vi "Begin.vi"(8 "error in":errorcluster) -> (0 "error out":errorcluster)   [LabVIEW 2016]
doc: "Called before other user functions, this VI is expected to open initial I/O refnums, load in file data, and do all program initialization. Notice that the <B>error out</B> terminal is simply used for data flow. Wiring it to other structures or subVIs ensures that this VI runs first."
uses:
  <vilib>/Rock Robotics/WPI/DriverStation/WPI_DriverStationRobotMode2.ctl
  <vilib>/Rock Robotics/WPI/Joystick/WPI_JoystickDeviceEnum.ctl
  <vilib>/Rock Robotics/SystemInterfaces/DIO/FPGA_DIOPWMChannel.ctl
  <vilib>/Rock Robotics/SystemInterfaces/AI/FPGA_AIChannel.ctl
  <vilib>/Rock Robotics/SystemInterfaces/DIO/FPGA_DIOChannel.ctl
  <vilib>/Rock Robotics/WPI/Solenoid/WPI_SolenoidChannel.ctl
  <vilib>/Rock Robotics/SystemInterfaces/spilib/spi_bus.ctl
  <vilib>/Rock Robotics/WPI/Solenoid/WPI_SolenoidValue.ctl
  <vilib>/Rock Robotics/WPI/SafetyOutput/WPI_SafetyOutputConfigMenu.ctl
  <vilib>/Rock Robotics/WPI/ThirdParty/CanMotor/TalonSRX/WPI_CANTalonSRX_APIControlMode.ctl
  <vilib>/Rock Robotics/SystemInterfaces/AI/FPGA_AIGyroChannel.ctl
  Robot Global Data.vi
  <vilib>/Rock Robotics/Network Tables/NT Write String Array.vi
  <vilib>/Rock Robotics/WPI/MotorControl/WPI_MotorControlOpen VictorSP.vi
  <vilib>/Rock Robotics/Network Tables/NT Write Number.vi
  <vilib>/Rock Robotics/WPI/Counter/WPI_CounterDigitalInputToDigitalSource.vi
  <vilib>/Rock Robotics/WPI/Solenoid/WPI_SolenoidOpenSingle.vi
  <vilib>/Rock Robotics/WPI/Solenoid/WPI_SolenoidOpenDouble.vi
  <vilib>/Rock Robotics/WPI/Gyro/WPI_GyroXRS450_SPI_Open.vi
  <vilib>/Rock Robotics/WPI/Solenoid/WPI_SolenoidSetEnum.vi
  <vilib>/Rock Robotics/WPI/RobotDrive/WPI_RobotDriveOpen4MotorWithExistingMotors.vi
  <vilib>/Rock Robotics/WPI/Gyro/WPI_GyroAnalogOpen.vi
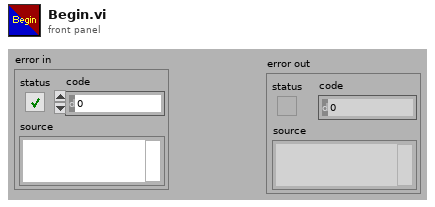
[diagram p1: front panel]
types:
  T1 = typedef "FPGA_AIGyroChannel.ctl" = enum8{"AI 0", "AI 1", "Invalid"}
  T2 = typedef "WPI_CANTalonSRX_APIControlMode.ctl" = enum8{"Percent VBus", "Speed", "Position", "Slave", "Unchanged / Invalid", "Voltage Compensation", "Current", "Motion Profile", "Motion Magic"}
  T3 = typedef "FPGA_DIOPWMChannel.ctl" = enum8{"PWM 0", "PWM 1", "PWM 2", "PWM 3", "PWM 4", "PWM 5", "PWM 6", "PWM 7", "PWM 8", "PWM 9", "PWM MXP 0", "PWM MXP 1", "PWM MXP 2", "PWM MXP 3", "PWM MXP 4", "PWM MXP 5", "PWM MXP 6", "PWM MXP 7", "PWM MXP 8", "PWM MXP 9", "Invalid"}
  T4 = typedef "WPI_SafetyOutputConfigMenu.ctl" = enum16{"Enable", "Disable"}
  T5 = typedef "WPI_SolenoidValue.ctl" = enum16{"Off", "On", "Forward", "Reverse"}
  T6 = typedef "spi_bus.ctl" = enum16{"SPI On-Board, CS0", "SPI On-Board, CS1", "SPI On-Board, CS2", "SPI On-Board, CS3", "SPI MXP", "Invalid"}
  T7 = typedef "WPI_SolenoidChannel.ctl" = enum8{"Solenoid 0", "Solenoid 1", "Solenoid 2", "Solenoid 3", "Solenoid 4", "Solenoid 5", "Solenoid 6", "Solenoid 7", "Invalid"}
  T8 = typedef "FPGA_DIOChannel.ctl" = enum8{"DIO 0", "DIO 1", "DIO 2", "DIO 3", "DIO 4", "DIO 5", "DIO 6", "DIO 7", "DIO 8", "DIO 9", "DIO MXP 0", "DIO MXP 1", "DIO MXP 2", "DIO MXP 3", "DIO MXP 4", "DIO MXP 5", "DIO MXP 6", "DIO MXP 7", "DIO MXP 8", "DIO MXP 9", "DIO MXP 10", "DIO MXP 11", "DIO MXP 12", "DIO MXP 13", "DIO MXP 14", "DIO MXP 15", "SPI Port CS1", "SPI Port CS2", "SPI Port CS3", "SPI Port MISO", "SPI Port MOSI", "Invalid"}
  T9 = typedef "FPGA_AIChannel.ctl" = enum8{"AI 0", "AI 1", "AI 2", "AI 3", "AI MXP 0", "AI MXP 1", "AI MXP 2", "AI MXP 3", "Invalid"}
  T10 = typedef "WPI_JoystickDeviceEnum.ctl" = enum16{"USB 0", "USB 1", "USB 2", "USB 3", "USB 4", "USB 5"}
  T11 = typedef "WPI_DriverStationRobotMode2.ctl" = enum16{"Autonomous Disabled", "Autonomous Enabled", "Teleop Disabled", "Teleop Enabled", "Disconnected", "Finish", "Test Disabled", "Test Enabled", "Emergency Stopped"}
  T12 = typedef "WPI_MotorControlDeviceRef.ctl" = cluster{"DeviceStatus":errorcluster, "Type":T13, "PWM":cluster{"PWM Channel":T3, "DeadBand":T14}, "CAN":cluster{"Device Number":u8, "SetOutput VI Ref":variant, "GetOutput VI Ref":variant, "Enable VI Ref":variant, "Disable VI Ref":variant, "Data":variant}, "Invert":bool}
  T13 = typedef "WPI_MotorControlType.ctl" = enum16{"PWM", "CAN"}
  T14 = typedef "WPI_PWMDeadband.ctl" = cluster{"Name":string, "maxPositivePwm":i32, "minPositivePwm":i32, "centerPwm":i32, "maxNegativePwm":i32, "minNegativePwm":i32, "angularRange":u16}
  T15 = typedef "WPI_PotentiometerDevRef.ctl" = cluster{"DevStatus":errorcluster, "Analog Channel":T9, "Invert Output":bool}
  T16 = typedef "WPI_DigitalInputDevRef.ctl" = cluster{"DevStatus":errorcluster, "DIO Channel":T8}
  T17 = typedef "WPI_JoystickDevRef.ctl" = cluster{"Device":T10}
  T18 = typedef "WPI_SolenoidDevRef.ctl" = cluster{"DevStatus":errorcluster, "Pneumatics Control Module":u8, "Forward Solenoid Channel":T7, "Reverse Solenoid Channel":T7}
  T19 = typedef "WPI_RobotDriveDevRef.ctl" = cluster{"DevStatus":errorcluster, "Motors[]":T12[], "Square Inputs":bool, "Max Output":dbl}
  T20 = typedef "FPGA_CounterEncoderSourceConvertionLVSourceType.ctl" = cluster{"DevStatus":errorcluster, "AnalogTriggerMode?":bool, "DigitalMode":cluster{"DIO Channel":T21}, "AnalogTriggerMode":cluster{"AnalogTriggerIndex":T22, "OutputType":T23}}
  T21 = typedef "FPGA_DIODigitalSourceChannel.ctl" = enum8{"DIO 0", "DIO 1", "DIO 2", "DIO 3", "DIO 4", "DIO 5", "DIO 6", "DIO 7", "DIO 8", "DIO 9", "DIO MXP 0", "DIO MXP 1", "DIO MXP 2", "DIO MXP 3", "DIO MXP 4", "DIO MXP 5", "DIO MXP 6", "DIO MXP 7", "DIO MXP 8", "DIO MXP 9", "DIO MXP 10", "DIO MXP 11", "DIO MXP 12", "DIO MXP 13", "DIO MXP 14", "DIO MXP 15", "Disabled"}
  T22 = typedef "FPGA_AnalogTriggerIndex.ctl" = enum8{"Trig 0", "Trig 1", "Trig 2", "Trig 3", "Trig 4", "Trig 5", "Trig 6", "Trig 7", "Invalid"}
  T23 = typedef "FPGA_AnalogTriggerOutType.ctl" = enum16{"InWindow", "TriggerState", "Rising", "Falling"}
  T24 = typedef "WPI_EncoderDevRef.ctl" = cluster{"DevStatus":errorcluster, "EncoderIndex":T25, "CounterIndex":T26, "DistancePerCount":dbl, "Decoding Type":T27}
  T25 = typedef "FPGA_EncoderIdx.ctl" = enum8{"Enc 0", "Enc 1", "Enc 2", "Enc 3", "Enc 4", "Enc 5", "Enc 6", "Enc 7", "Invalid"}
  T26 = typedef "FPGA_CounterCtrSystemIndex.ctl" = enum8{"Ctr 0", "Ctr 1", "Ctr 2", "Ctr 3", "Ctr 4", "Ctr 5", "Ctr 6", "Ctr 7", "Invalid"}
  T27 = typedef "WPI_EncoderType.ctl" = enum16{"1x", "2x", "4x"}
  T28 = typedef "WPI_GyroDevRef.ctl" = cluster{"DevStatus":errorcluster, "Analog Channel":T9, "Offset":dbl, "Gain (VoltsPerDegree/Second)":dbl, "Gyro Type":enum16{"Analog", "XRS450"}, "Handle":i32, "SPI Bus":T6, "Device Found":bool, "Sample Rate":dbl, "Calibrate On Open":bool}
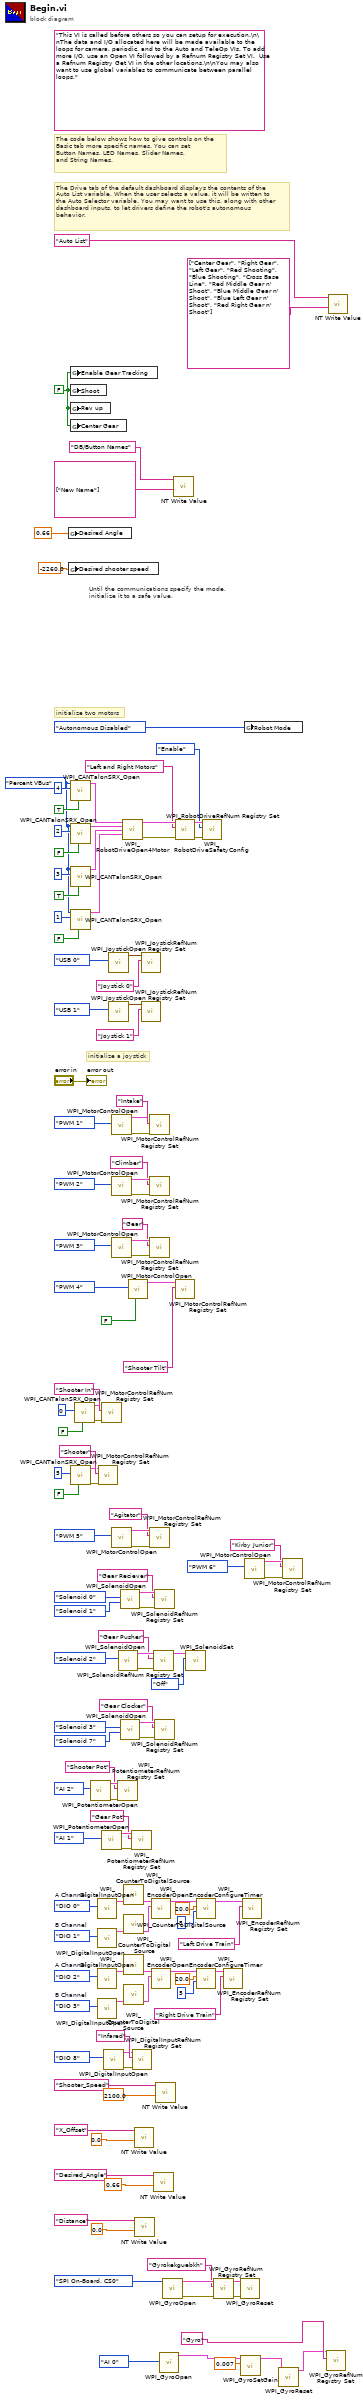
[diagram p0: block diagram]
diagram:
  w8 = WPI_CANTalonSRX_APIControlMode."Percent VBus" ("Control Mode")
  w99 = FPGA_DIOChannel."DIO 3"  # B Channel
  w98 = FPGA_DIOChannel."DIO 2"  # A Channel
  w106 = FPGA_DIOChannel."DIO 1"  # B Channel
  w105 = FPGA_DIOChannel."DIO 0"  # A Channel
  w117 = FALSE
  (unwired) "This VI is called before others so you can setup for execution.\n\nThe data and I/O allocated here will be made available to the loops for camera, periodic, and to the Auto and TeleOp VIs. To add more I/O, use an Open VI followed by a Refnum Registry Set VI.  Use a Refnum Registry Get VI in the other locations.\n\nYou may also want to use global variables to communicate between parallel loops."
  # "initialize two motors"
  # "The Drive tab of the default dashboard displays the contents of the\nAuto List variable. When the user selects a value, it will be written to\nthe Auto Selector variable. You may want to use this, along with other\ndashboard inputs, to let drivers define the robot's autonomous\nbehavior."
  # "The code below shows how to give controls on the\nBasic tab more specific names. You can set\nButton Names, LED Names, Slider Names,\nand String Names."
  # "initialize a joystick"
  # "Until the communications specify the mode,\ninitialize it to a safe value."
  n1 = global write "Robot Global Data.vi" "Desired Angle"(0.66) -> ()
  n2 = global write "Robot Global Data.vi" "Desired shooter speed"(-2260.0) -> ()
  n3 = global write "Robot Global Data.vi" "Enable Gear Tracking"(w117) -> ()
  n4 = global write "Robot Global Data.vi" "Shoot"(w117) -> ()
  n5 = global write "Robot Global Data.vi" "Rev up"(w117) -> ()
  n6 = global write "Robot Global Data.vi" "Center Gear"(w117) -> ()
  n7 = call <vilib>:"WPI_CANTalonSRX_Open.vi"("Invert"=TRUE, "Device Number"=u8 4, "Control Mode"=w8) -> ("CAN Talon SRX Ref"=w21:T12)  [unwired: 7 in, 1 out]
  n8 = call <vilib>:"WPI_CANTalonSRX_Open.vi"("Invert"=FALSE, "Device Number"=u8 2, "Control Mode"=w8) -> ("CAN Talon SRX Ref"=w22:T12)  [unwired: 7 in, 1 out]
  n9 = call <vilib>:"WPI_CANTalonSRX_Open.vi"("Invert"=TRUE, "Device Number"=u8 3, "Control Mode"=w8) -> ("CAN Talon SRX Ref"=w23:T12)  [unwired: 7 in, 1 out]
  n10 = call <vilib>:"WPI_CANTalonSRX_Open.vi"("Invert"=FALSE, "Device Number"=u8 1, "Control Mode"=w8) -> ("CAN Talon SRX Ref"=w24:T12)  [unwired: 7 in, 1 out]
  n11 = call <vilib>:"WPI_CANTalonSRX_Open.vi"("Invert"=FALSE, "Device Number"=u8 5) -> ("error out"=w49:errorcluster, "CAN Talon SRX Ref"=w50:T12)  [unwired: 8 in]
  n12 = call <vilib>:"WPI_CANTalonSRX_Open.vi"("Invert"=FALSE, "Device Number"=u8 0) -> ("error out"=w51:errorcluster, "CAN Talon SRX Ref"=w52:T12)  [unwired: 8 in]
  n13 = call <vilib>:"WPI_PotentiometerOpen.vi"("Analog Channel"=FPGA_AIChannel."AI 2") -> ("error out"=w64:errorcluster, "PotDevRef"=w108:T15)  [unwired: 9 in]
  n14 = call <vilib>:"WPI_DigitalInputOpen.vi"("DIO Channel"=w105) -> ("DigitalInputDevRef"=w102:T16)  [unwired: 1 in, 9 out]
  n15 = call <vilib>:"WPI_DigitalInputOpen.vi"("DIO Channel"=w106) -> ("DigitalInputDevRef"=w103:T16)  [unwired: 1 in, 9 out]
  n16 = call <vilib>:"WPI_DigitalInputOpen.vi"("DIO Channel"=w98) -> ("DigitalInputDevRef"=w95:T16)  [unwired: 1 in, 9 out]
  n17 = call <vilib>:"WPI_DigitalInputOpen.vi"("DIO Channel"=w99) -> ("DigitalInputDevRef"=w96:T16)  [unwired: 1 in, 9 out]
  n18 = call <vilib>:"WPI_MotorControlRefNum Registry Set.vi"("error in (no error)"=w49, "refnum name"="Shooter", "MotorControlDevRef"=w50) -> ()  [unwired: 7 in, 2 out]
  n19 = call <vilib>:"WPI_MotorControlRefNum Registry Set.vi"("error in (no error)"=w51, "refnum name"="Shooter In", "MotorControlDevRef"=w52) -> ()  [unwired: 7 in, 2 out]
  n20 = call <vilib>:"WPI_PotentiometerOpen.vi"("Analog Channel"=FPGA_AIChannel."AI 1") -> ("error out"=w63:errorcluster, "PotDevRef"=w91:T15)  [unwired: 9 in]
  n21 = call <vilib>:"WPI_DigitalInputOpen.vi"("DIO Channel"=FPGA_DIOChannel."DIO 8") -> ("error out"=w62:errorcluster, "DigitalInputDevRef"=w75:T16)  [unwired: 9 in]
  n22 = call <vilib>:"WPI_JoystickOpen.vi"("JoystickDevice"=WPI_JoystickDeviceEnum."USB 0") -> ("JoystickDevRef"=w136:T17)  [unwired: 10 in]
  n23 = call <vilib>:"WPI_JoystickOpen.vi"("JoystickDevice"=WPI_JoystickDeviceEnum."USB 1") -> ("JoystickDevRef"=w128:T17)  [unwired: 10 in]
  n24 = call-poly <vilib>:"WPI_MotorControlOpen.vi"("PWM Channel"=FPGA_DIOPWMChannel."PWM 1") -> ("error out"=w17:errorcluster, "MotorControlDeviceRef"=w16:T12)  [unwired: 9 in]
  n25 = call-poly <vilib>:"WPI_MotorControlOpen.vi"("PWM Channel"=FPGA_DIOPWMChannel."PWM 2") -> ("error out"=w70:errorcluster, "MotorControlDeviceRef"=w126:T12)  [unwired: 9 in]
  n26 = call-poly <vilib>:"WPI_MotorControlOpen.vi"("PWM Channel"=FPGA_DIOPWMChannel."PWM 3") -> ("error out"=w69:errorcluster, "MotorControlDeviceRef"=w123:T12)  [unwired: 9 in]
  n27 = call-poly <vilib>:"WPI_MotorControlOpen.vi"("PWM Channel"=FPGA_DIOPWMChannel."PWM 5") -> ("error out"=w68:errorcluster, "MotorControlDeviceRef"=w74:T12)  [unwired: 9 in]
  n28 = call <vilib>:"WPI_PotentiometerRefNum Registry Set.vi"("error in (no error)"=w64, "refnum name"="Shooter Pot", "PotDevRef"=w108) -> ()  [unwired: 7 in, 2 out]
  n29 = call-poly <vilib>:"WPI_SolenoidOpen.vi"("Solenoid Channel"=WPI_SolenoidChannel."Solenoid 2") -> ("error out"=w66:errorcluster, "SolenoidDevRef"=w85:T18)  [unwired: 9 in]
  n30 = call-poly <vilib>:"WPI_SolenoidOpen.vi"("Reverse Solenoid Channel"=WPI_SolenoidChannel."Solenoid 1", "Forward Solenoid Channel"=WPI_SolenoidChannel."Solenoid 0" ("Solenoid Channel")) -> ("error out"=w67:errorcluster, "SolenoidDevRef"=w88:T18)  [unwired: 8 in]
  n31 = call-poly <vilib>:"WPI_SolenoidOpen.vi"("Reverse Solenoid Channel"=WPI_SolenoidChannel."Solenoid 7", "Forward Solenoid Channel"=WPI_SolenoidChannel."Solenoid 3" ("Solenoid Channel")) -> ("error out"=w65:errorcluster, "SolenoidDevRef"=w82:T18)  [unwired: 8 in]
  n32 = call-poly <vilib>:"WPI_RobotDriveOpen4Motor.vi"("Rear Left Motor Dev Ref"=w21, "Rear Right Motor Dev Ref"=w22, "Front Left Motor Dev Ref"=w23, "Front Right Motor Dev Ref"=w24) -> ("RobotDriveDevRef"=w37:T19, "error out"=w35:errorcluster)  [unwired: 10 in]
  n33 = call-poly <vilib>:"WPI_CounterToDigitalSource.vi"("DigitalInputDevRef"=w102) -> ("Digital Source"=w101:T20)  [unwired: 6 out]
  n34 = call-poly <vilib>:"WPI_CounterToDigitalSource.vi"("DigitalInputDevRef"=w103) -> ("Digital Source"=w104:T20)  [unwired: 6 out]
  n35 = call-poly <vilib>:"WPI_CounterToDigitalSource.vi"("DigitalInputDevRef"=w95) -> ("Digital Source"=w94:T20)  [unwired: 6 out]
  n36 = call-poly <vilib>:"WPI_CounterToDigitalSource.vi"("DigitalInputDevRef"=w96) -> ("Digital Source"=w97:T20)  [unwired: 6 out]
  n37 = call-poly <vilib>:"WPI_MotorControlOpen.vi"("Invert"=FALSE, "PWM Channel"=FPGA_DIOPWMChannel."PWM 4") -> ("MotorControlDeviceRef"=w13:T12)  [unwired: 8 in, 1 out]
  n38 = call <vilib>:"WPI_PotentiometerRefNum Registry Set.vi"("error in (no error)"=w63, "refnum name"="Gear Pot", "PotDevRef"=w91) -> ()  [unwired: 7 in, 2 out]
  n39 = call <vilib>:"WPI_DigitalInputRefNum Registry Set.vi"("error in (no error)"=w62, "refnum name"="Infared", "DigitalInputDevRef"=w75) -> ()  [unwired: 7 in, 2 out]
  n40 = call-poly <vilib>:"NT Write Value.vi"("Numeric"=0.0, "Name"="X_Offset") -> ()  [unwired: 9 in, 1 out]
  n41 = call-poly <vilib>:"NT Write Value.vi"("Numeric"=0.0, "Name"="Distance") -> ()  [unwired: 9 in, 1 out]
  n42 = call <vilib>:"WPI_JoystickRefNum Registry Set.vi"("refnum name"="Joystick 0", "JoystickDevRef"=w136) -> ()  [unwired: 8 in, 2 out]
  n43 = call <vilib>:"WPI_JoystickRefNum Registry Set.vi"("refnum name"="Joystick 1", "JoystickDevRef"=w128) -> ()  [unwired: 8 in, 2 out]
  n44 = call <vilib>:"WPI_MotorControlRefNum Registry Set.vi"("error in (no error)"=w17, "refnum name"="Intake", "MotorControlDevRef"=w16) -> ()  [unwired: 7 in, 2 out]
  n45 = call <vilib>:"WPI_MotorControlRefNum Registry Set.vi"("error in (no error)"=w70, "refnum name"="Climber", "MotorControlDevRef"=w126) -> ()  [unwired: 7 in, 2 out]
  n46 = call <vilib>:"WPI_MotorControlRefNum Registry Set.vi"("error in (no error)"=w69, "refnum name"="Gear", "MotorControlDevRef"=w123) -> ()  [unwired: 7 in, 2 out]
  n47 = call <vilib>:"WPI_MotorControlRefNum Registry Set.vi"("error in (no error)"=w68, "refnum name"="Agitator", "MotorControlDevRef"=w74) -> ()  [unwired: 7 in, 2 out]
  n48 = call <vilib>:"WPI_EncoderOpen.vi"("BSource"=w104, "ASource"=w101) -> ("EncoderDevRef"=w39:T24)  [unwired: 6 in, 3 out]
  n49 = call <vilib>:"WPI_EncoderOpen.vi"("BSource"=w97, "ASource"=w94) -> ("EncoderDevRef"=w43:T24)  [unwired: 6 in, 3 out]
  n50 = call <vilib>:"WPI_SolenoidRefNum Registry Set.vi"("error in (no error)"=w66, "refnum name"="Gear Pusher", "SolenoidDevRef"=w85) -> ("SolenoidDevRef"=w57:T18)  [unwired: 7 in, 1 out]
  n51 = call-poly <vilib>:"NT Write Value.vi"("Numeric"=0.66, "Name"="Desired_Angle") -> ()  [unwired: 9 in, 1 out]
  n52 = call <vilib>:"WPI_SolenoidRefNum Registry Set.vi"("error in (no error)"=w67, "refnum name"="Gear Reciever", "SolenoidDevRef"=w88) -> ()  [unwired: 7 in, 2 out]
  n53 = call <vilib>:"WPI_SolenoidRefNum Registry Set.vi"("error in (no error)"=w65, "refnum name"="Gear Clocker", "SolenoidDevRef"=w82) -> ()  [unwired: 7 in, 2 out]
  n54 = call-poly <vilib>:"NT Write Value.vi"("Numeric"=2100.0, "Name"="Shooter_Speed") -> ()  [unwired: 9 in, 1 out]
  n55 = call-poly <vilib>:"WPI_GyroOpen.vi"("Analog Channel"=FPGA_AIGyroChannel."AI 0") -> ("GyroDevRef"=w4:T28)  [unwired: 8 in, 2 out]
  n56 = call-poly <vilib>:"WPI_GyroOpen.vi"("SPI Bus"=spi_bus."SPI On-Board, CS0") -> ("error out"=w59:errorcluster, "GyroDevRef"=w60:T28)  [unwired: 9 in]
  n57 = call-poly <vilib>:"NT Write Value.vi"("String Array"=string[] ["New Name"], "Name"="DB/Button Names") -> ()  [unwired: 9 in, 1 out]
  n58 = call <vilib>:"WPI_RobotDriveRefNum Registry Set.vi"("error in (no error)"=w35, "refnum name"="Left and Right Motors", "RobotDriveDevRef"=w37) -> ("error out"=w20:errorcluster, "RobotDriveDevRef"=w34:T19)  [unwired: 1 in, 6 out]
  n59 = call <vilib>:"WPI_MotorControlRefNum Registry Set.vi"("refnum name"="Shooter Tilt", "MotorControlDevRef"=w13) -> ()  [unwired: 8 in, 2 out]
  n60 = call-poly <vilib>:"WPI_SolenoidSet.vi"("Value"=WPI_SolenoidValue."Off", "SolenoidDevRef"=w57) -> ()  [unwired: 8 in, 2 out]
  n61 = call <vilib>:"WPI_EncoderConfigureTimer.vi"("Number Samples to Average"=u8 5, "Minimum Rate"=20.0, "EncoderDevRef"=w39) -> ("EncoderDevRef"=w38:T24)  [unwired: 7 in, 1 out]
  n62 = call <vilib>:"WPI_EncoderConfigureTimer.vi"("Number Samples to Average"=u8 5, "Minimum Rate"=20.0, "EncoderDevRef"=w43) -> ("EncoderDevRef"=w42:T24)  [unwired: 7 in, 1 out]
  n63 = call <vilib>:"WPI_RobotDriveSafetyConfig.vi"("error in (no error)"=w20, "mode"=WPI_SafetyOutputConfigMenu."Enable", "RobotDriveDevRef"=w34) -> ()  [unwired: 7 in, 2 out]
  n64 = call <vilib>:"WPI_GyroRefNum Registry Set.vi"("error in (no error)"=w59, "refnum name"="Gyrokekguebkh", "GyroDevRef"=w60) -> ("error out"=w55:errorcluster, "GyroDevRef"=w54:T28)  [unwired: 7 in]
  n65 = call <vilib>:"WPI_EncoderRefNum Registry Set.vi"("refnum name"="Right Drive Train", "EncoderDevRef"=w42) -> ()  [unwired: 8 in, 2 out]
  n66 = call <vilib>:"WPI_GyroReset.vi"("error in"=w55, "GyroDevRef"=w54) -> ()  [unwired: 8 in, 2 out]
  n67 = call <vilib>:"WPI_GyroSetGain.vi"("Gain (VoltsPerDegree/Second)"=0.007, "GyroDevRef"=w4) -> ("GyroDevRef"=w2:T28)  [unwired: 8 in, 1 out]
  n68 = call <vilib>:"WPI_EncoderRefNum Registry Set.vi"("refnum name"="Left Drive Train", "EncoderDevRef"=w38) -> ()  [unwired: 8 in, 2 out]
  n69 = global write "Robot Global Data.vi" "Robot Mode"(WPI_DriverStationRobotMode2."Autonomous Disabled" ("Robot Mode")) -> ()
  n70 = call-poly <vilib>:"WPI_MotorControlOpen.vi"("PWM Channel"=FPGA_DIOPWMChannel."PWM 6") -> ("error out"=w9:errorcluster, "MotorControlDeviceRef"=w12:T12)  [unwired: 9 in]
  n71 = call <vilib>:"WPI_GyroReset.vi"("GyroDevRef"=w2) -> ("GyroDevRef"=w1:T28)  [unwired: 9 in, 1 out]
  n72 = call <vilib>:"WPI_MotorControlRefNum Registry Set.vi"("error in (no error)"=w9, "refnum name"="Kirby Junior", "MotorControlDevRef"=w12) -> ()  [unwired: 7 in, 2 out]
  n73 = call <vilib>:"WPI_GyroRefNum Registry Set.vi"("refnum name"="Gyro", "GyroDevRef"=w1) -> ()  [unwired: 8 in, 2 out]
  n74 = call-poly <vilib>:"NT Write Value.vi"("String Array"=string[] ["Center Gear", "Right Gear", "Left Gear", "Red Shooting", "Blue Shooting", "Cross Base Line", "Red Middle Gear n' Shoot", "Blue Middle Gear n' Shoot", "Blue Left Gear n' Shoot", "Red Right Gear n' Shoot"], "Name"="Auto List") -> ()  [unwired: 9 in, 1 out]
  "error out" <- "error in"
